vi "NodeRefToNodeInfo.vi"(8 "error in (no error)":errorcluster, 11 "Node":T1) -> (0 "error out":errorcluster, 2 "NodeInfo":T2, 3 "Node":T1)   [LabVIEW 2020, in "NI_VS Workspace ExecutionAPI.lvlib"]
uses:
  <vilib>/NI VeriStand/Execution/Workspace/NI_VS Workspace ExecutionAPI.lvlib
  <vilib>/NI VeriStand/Execution/Workspace/NodeInfo.ctl
  <vilib>/NI VeriStand/Execution/Workspace/Waveform Data Type.ctl
  <vilib>/NI VeriStand/Execution/Workspace/NodeObj.ctl
  NationalInstruments.VeriStand.ClientAPI
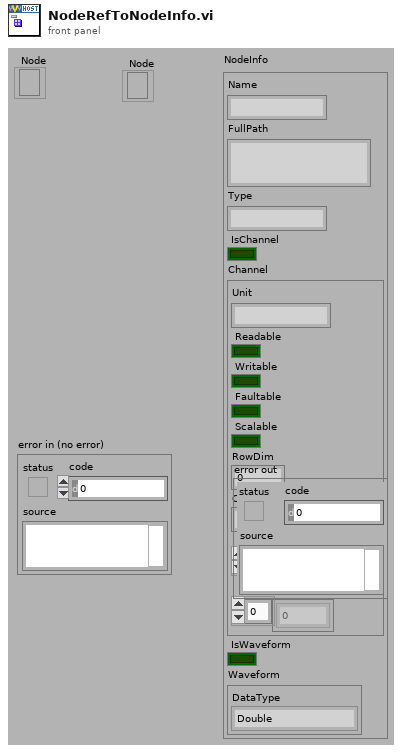
[diagram p1: front panel]
types:
  T1 = typedef "NI_VS Workspace ExecutionAPI.lvlib/NodeObj.ctl" = refnum<k24>
  T2 = typedef "NI_VS Workspace ExecutionAPI.lvlib/NodeInfo.ctl" = cluster{"Name":string, "FullPath":string, "Type":string, "IsChannel":bool, "Channel":cluster{"Unit":string, "Readable":bool, "Writable":bool, "Faultable":bool, "Scalable":bool, "RowDim":u32, "ColumnDim":u32, "Value Table Names":string[], "Value Table Values":dbl[]}, "IsWaveform":bool, "Waveform":cluster{"DataType":T3}}
  T3 = typedef "NI_VS Workspace ExecutionAPI.lvlib/Waveform Data Type.ctl" = enum16{"Double", "ComplexDouble"}
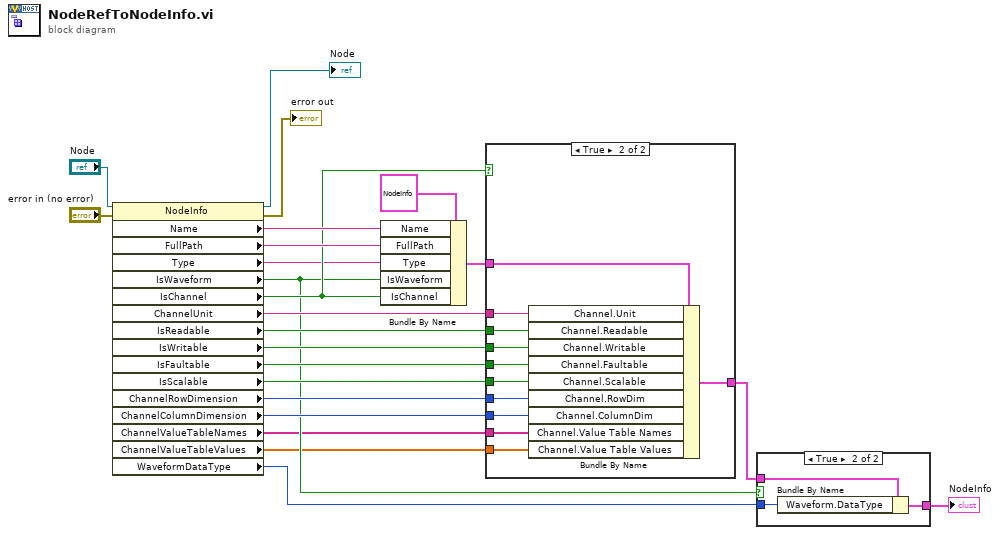
[diagram p0: block diagram]
diagram:
  n1 = property class="NodeInfo"(reference="Node", error in="error in (no error)") -> (reference out=→"Node":T1, error out=→"error out":errorcluster, "Name"=w23:string, "FullPath"=w22:string, "Type"=w9:string, "IsWaveform"=w4:bool, "IsChannel"=w10:bool, "ChannelUnit"=w20:string, "IsReadable"=w19:bool, "IsWritable"=w18:bool, "IsFaultable"=w17:bool, "IsScalable"=w16:bool, "ChannelRowDimension"=w8:u32, "ChannelColumnDimension"=w7:u32, "ChannelValueTableNames"=w2:string[], "ChannelValueTableValues"=w1:dbl[], "WaveformDataType"=w3:i32)
  n2 = Bundle By Name(cluster=T2 {"Name"="", "FullPath"="", "Type"="", "IsChannel"=FALSE, "Channel"={"Unit"="", "Readable"=FALSE, "Writable"=FALSE, "Faultable"=FALSE, "Scalable"=FALSE, "RowDim"=0, "ColumnDim"=0, "Value Table Names"=[], "Value Table Values"=[]}, "IsWaveform"=FALSE, "Waveform"={"DataType"=enum."Double"}} ("NodeInfo"), "Name"=w23, "FullPath"=w22, "Type"=w9, "IsWaveform"=w4, "IsChannel"=w10) -> (w21:T2)
  n3 = case shown="True" w10 {
    tunnel: w21 -> [w24 w35]
    tunnel: w20 -> [_ w34]
    tunnel: w19 -> [_ w33]
    tunnel: w18 -> [_ w32]
    tunnel: w17 -> [_ w31]
    tunnel: w16 -> [_ w30]
    tunnel: [w24 w29] -> w6
    tunnel: w8 -> [_ w28]
    tunnel: w7 -> [_ w27]
    tunnel: w2 -> [_ w26]
    tunnel: w1 -> [_ w25]
    frame False {
    }
    frame True {
      n4 = Bundle By Name(cluster=w35, "Channel.Unit"=w34, "Channel.Readable"=w33, "Channel.Writable"=w32, "Channel.Faultable"=w31, "Channel.Scalable"=w30, "Channel.RowDim"=w28, "Channel.ColumnDim"=w27, "Channel.Value Table Names"=w26, "Channel.Value Table Values"=w25) -> (w29:T2)
    }
  }
  n5 = case shown="True" w4 {
    tunnel: w6 -> [w36 w39]
    tunnel: w3 -> [_ w37]
    tunnel: [w36 w38] -> w5
    frame False {
    }
    frame True {
      n6 = Bundle By Name(cluster=w39, "Waveform.DataType"=w37) -> (w38:T2)
    }
  }
  "NodeInfo" <- w5
